vi "queues2.vi"() -> ()   [LabVIEW 2019]
doc: "This is the first of two demos using Queues. In this demo, one While loop takes the same role as the first loop in the Notifier example, whilst the second While loop plots data. Here, however, the Wait period in the second (consumer) loop is longer than the producer, and so data builds up over time. Because these are using a Queue, the data is not lost - it merely becomes backlogged."
panel:
  out "Consumer":i32
  out "Producer":i32
  in  "stop":bool
  out "Waveform Chart":dbl(graph)
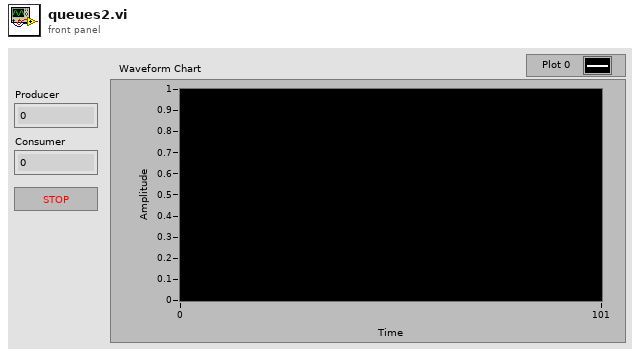
[diagram p1: front panel]
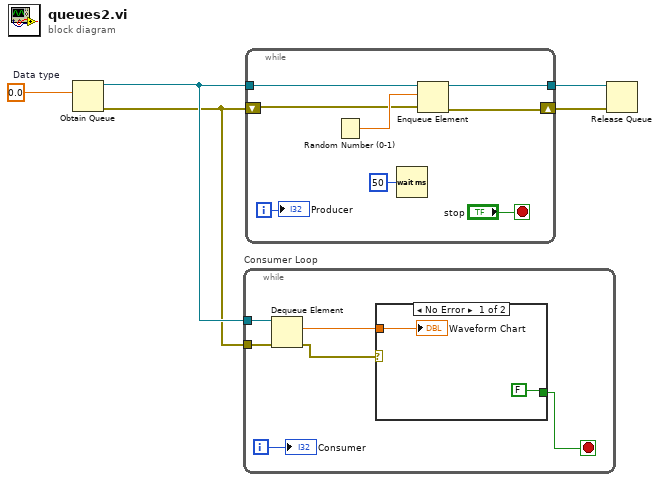
[diagram p0: block diagram]
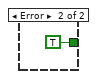
[diagram p2: hidden frame]
diagram:
  w4 = 0.0  # Data type
  n1 = Obtain Queue(element data type=w4) -> (queue out=w5:refnum<queue>, error out=w1:errorcluster)  [unwired: 4 in, 1 out]
  n2 = while "Consumer Loop" {
    tunnel: w5 -> [w11]
    tunnel: w1 -> [w6]
    i -> [w10]
    stop <- w7 stop-if-true
    n3 = Dequeue Element(queue=w11, error in (no error)=w6) -> (element=w8:dbl, error out=w9:errorcluster)  [unwired: 1 in, 2 out]
    n4 = case shown="No Error" w9 {
      tunnel: w8 -> [w13 _]
      tunnel: [FALSE TRUE] -> w7
      frame No Error {
        "Waveform Chart" <- w13
      }
      frame Error {
      }
    }
    "Consumer" <- w10
  }
  n5 = while {
    tunnel: w5 -> [w22]
    shift-right: [w16] -> w2
    shift-left: w1 -> [w17]
    tunnel: [w15] -> w3
    i -> [w20]
    stop <- "stop" stop-if-true
    n6 = Random Number (0-1)() -> (number: 0 to 1=w18:dbl)
    n7 = Wait (ms)(milliseconds to wait=u32 50) -> ()  [unwired: 1 out]
    n8 = Enqueue Element(queue=w22, element=w18, error in (no error)=w17) -> (queue out=w15:refnum<queue>, error out=w16:errorcluster)  [unwired: 1 in, 1 out]
    "Producer" <- w20
  }
  n9 = Release Queue(queue=w3, error in (no error)=w2) -> ()  [unwired: 1 in, 3 out]
